vi "recipeScript setNewFilePath.vi"(7 "newfilePath":path, 8 "error in (no error)":errorcluster, 11 "filePathRefnum in":refnum<vi>) -> (0 "error out":errorcluster, 1 "valid":bool, 3 "filePathRefnum out":refnum<vi>)   [LabVIEW 2018]
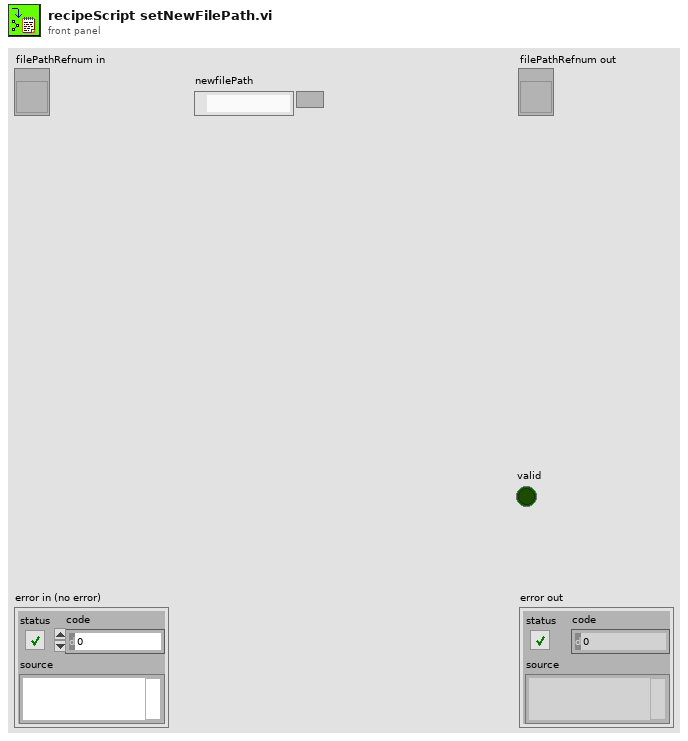
[diagram p1: front panel]
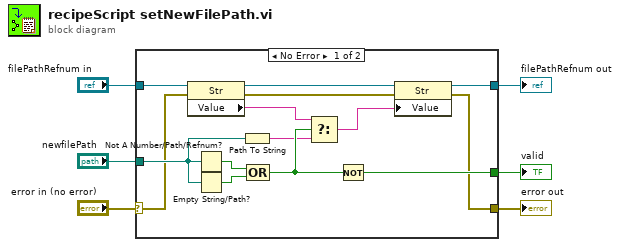
[diagram p0: block diagram]
diagram:
  n1 = case shown="No Error" "error in (no error)" {
    selector: "error in (no error)" -> [w9 w22]
    tunnel: "filePathRefnum in" -> [w20 w21]
    tunnel: [w15 _] -> w5
    tunnel: "newfilePath" -> [w14 _]
    tunnel: [w8 w22] -> w2
    tunnel: [w7 w21] -> w1
    frame No Error {
      n2 = property class="Str"(reference=w20, error in=w9) -> (reference out=w12:refnum<vi>, error out=w10:errorcluster, "Value"=w17:string)
      n3 = Not A Number/Path/Refnum?(number/path/refnum=w14) -> (NaN/Path/Refnum?=w19:bool)
      n4 = Empty String/Path?(string/path=w14) -> (empty?=w18:bool)
      n5 = Path To String(path=w14) -> (string=w13:string)
      n6 = Compound Arithmetic op=OR(w19, w18) -> (w16:bool)
      n7 = Select(t=w17, s=w16, f=w13) -> (s? t:f=w11:string)
      n8 = Not(x=w16) -> (.not. x?=w15:bool)
      n9 = property class="Str"(reference=w12, error in=w10, "Value"=w11) -> (reference out=w7:refnum<vi>, error out=w8:errorcluster)
    }
    frame Error {
    }
  }
  "error out" <- w2
  "valid" <- w5
  "filePathRefnum out" <- w1
